vi "2.Gamepad.vi"() -> ()   [LabVIEW 2011]
doc: "This VI show how to use the basic functions in the Input Device palette. It will show information about all the joysticks, keyboards and mice attached to the system (number of axes, buttons, pov, and the name). It will also give the current information for the first joystick attached to the system (location and button pressed). The current information for the first keyboard and mouse will also be displayed."
uses:
  <vilib>/Utility/inputDevices.llb/closeJoystick.vi
  <vilib>/Utility/inputDevices.llb/joystickAcquire.vi
panel:
  out "Motor (scaled)":u64
  out "Steer (scaled)":i32
  in  "?":enum32{"Control", "Check Control"}(tab)
  in  "Steering":u8(slide)=128 scale=0.0..255.0
  in  "Motor Speed":u8(slide)=128 scale=0.0..255.0
  in  "Destination Id":u8=7
  in  "Control Mode":enum16{"Manual", "GamePad"}(ring)
  out "WriteSF Error":errorcluster
  out "OpenSF Error":errorcluster
  out "Y-axis":i32
  out "X-axis":i32
  out "Button 12":bool
  out "Button 13":bool
  out "Button 14":bool
  out "Button 15":bool
  out "X-axis":i32
  out "Y-axis":i32
  out "Value":i32
  out "Button 10":bool
  out "Button 11":bool
  out "Button 5":bool
  out "Button 6":bool
  out "POV":i32
  in  "Message":string="LabVIEW was unable\nto detect a joystick."
  in  "Button":string="Continue"
  # "Left"
  # "Right"
  # "Full Forward"
  # "Full Rverse"
  # "Left Top"
  # "Right Top"
  # "Left Buttom"
  # "Right Buttom"
  # "8-way D-pad"
  # "Left Joystick"
  # "Right Joystick"
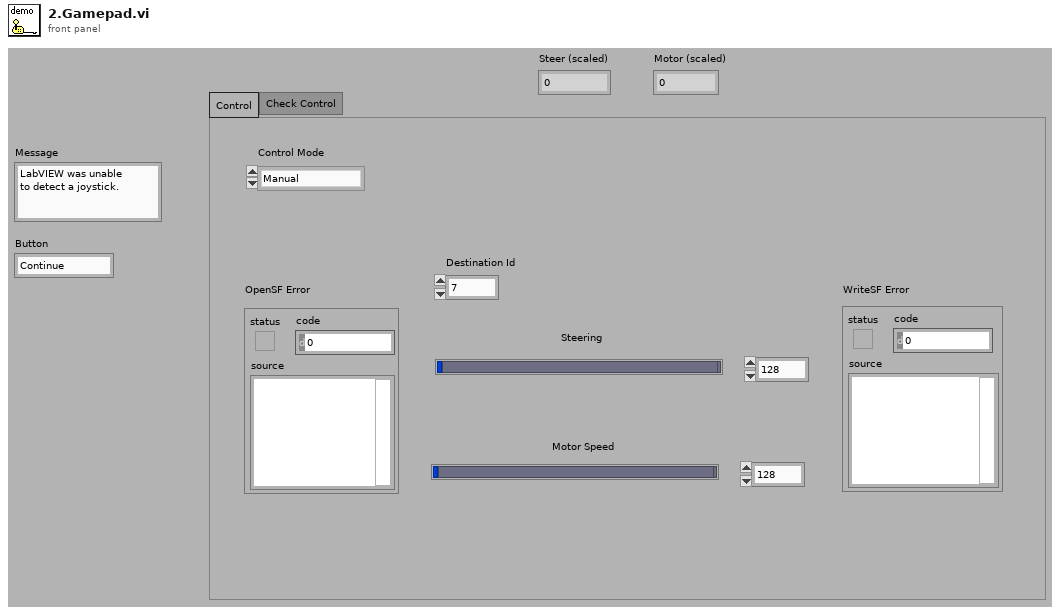
[diagram p1: front panel]
types:
  T1 = cluster{"X axis":i32, "Y axis":i32, "Z axis":i32, "X axis rotation":i32, "Y axis rotation":i32, "Z axis rotation":i32, "U axis":i32, "V axis":i32}
  T2 = cluster{"button 1":bool, "button 2":bool, "button 3":bool, "button 4":bool, "button 5":bool, "button 6":bool, "button 7":bool, "button 8":bool, "button 9":bool, "button 10":bool, "button 11":bool, "button 12":bool, "button 13":bool, "button 14":bool, "button 15":bool, "button 16":bool, "button 17":bool, "button 18":bool, "button 19":bool, "button 20":bool, "button 21":bool, "button 22":bool, "button 23":bool, "button 24":bool, "button 25":bool, "button 26":bool, "button 27":bool, "button 28":bool, "button 29":bool, "button 30":bool, "button 31":bool, "button 32":bool}
  T3 = cluster{"pov 1":i32, "pov 2":i32, "pov 3":i32, "pov 4":i32}
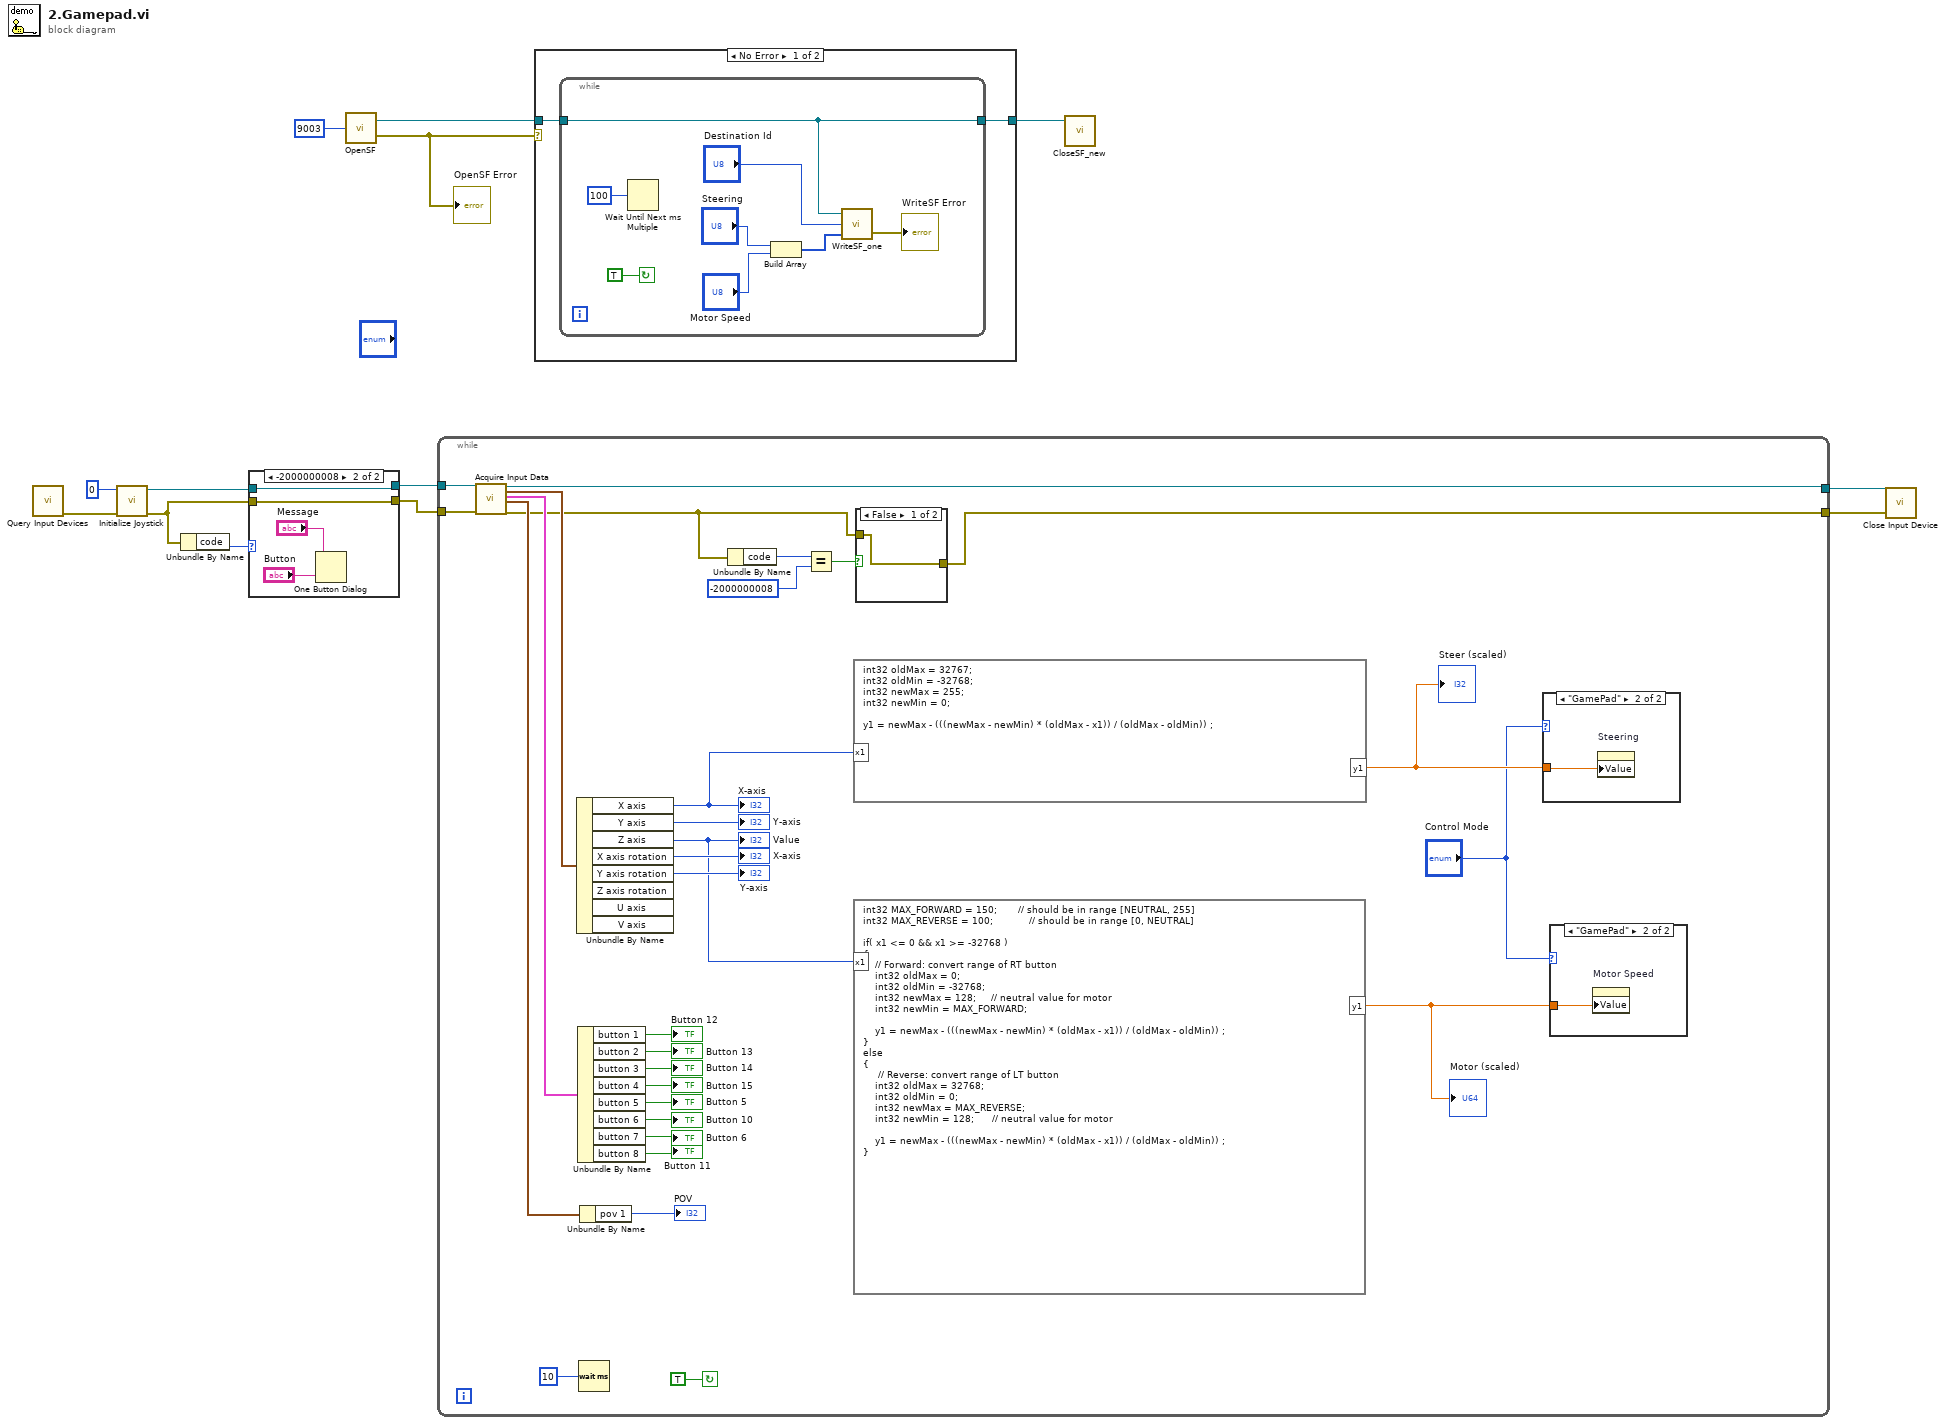
[diagram p0: block diagram]
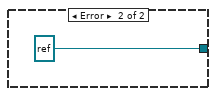
[diagram p2: hidden frame]
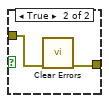
[diagram p6: hidden frame]
diagram:
  n1 = call <vilib>:"Query Input Devices.vi"() -> ("error out"=w13:errorcluster)  [unwired: 1 in, 10 out]
  n2 = call <vilib>:"Initialize Joystick.vi"("error in (no error)"=w13, "device index"=0) -> ("error out"=w7:errorcluster, "device ID"=w8:refnum<k1>)  [unwired: 8 out]
  n3 = Unbundle By Name(w7) -> ("code"=w9:i32)
  n4 = case shown="-2000000008" w9 {
    tunnel: w7 -> [w15 w17]
    tunnel: [w15 w17] -> w6
    tunnel: w8 -> [w14 w16]
    tunnel: [w14 w16] -> w5
    frame 0, Default {
    }
    frame -2000000008 {
      n5 = One Button Dialog(message="Message", button name ("OK")="Button") -> ()  [unwired: 1 out]
    }
  }
  n6 = call "OpenSF.vi"("Port number"=u16 9003 ("Port number\nactuators")) -> ("connection ID"=w2:refnum<k5>, "Error out"=w3:errorcluster)
  "OpenSF Error" <- w3
  n7 = while {
    tunnel: [w39] -> w11
    tunnel: [w43] -> w12
    tunnel: w6 -> [w37]
    tunnel: w5 -> [w36]
    stop <- TRUE continue-if-true
    n8 = call-poly <vilib>:"Acquire Input Data.vi"("device ID"=w36, "error in (no error)"=w37) -> ("device ID"=w43:refnum<k1>, "axis info"=w49:T1, "button info"=w47:T2, "direction info"=w46:T3, "error out"=w38:errorcluster)  [unwired: 13 out]
    n9 = Unbundle By Name(w49) -> ("X axis"=w26:i32, "Y axis"=→"Y-axis":i32, "Z axis"=w20:i32, "X axis rotation"=→"X-axis":i32, "Y axis rotation"=→"Y-axis":i32)  [unwired: 3 out]
    "X-axis" <- w26
    "Value" <- w20
    n10 = Unbundle By Name(w47) -> ("button 1"=→"Button 12":bool, "button 2"=→"Button 13":bool, "button 3"=→"Button 14":bool, "button 4"=→"Button 15":bool, "button 5"=→"Button 5":bool, "button 6"=→"Button 10":bool, "button 7"=→"Button 6":bool, "button 8"=→"Button 11":bool)
    n11 = Wait (ms)(milliseconds to wait=u32 10) -> ()  [unwired: 1 out]
    n12 = Unbundle By Name(w46) -> ("pov 1"=→"POV":i32)
    n13 = Unbundle By Name(w38) -> ("code"=w42:i32)
    n14 = Equal?(x=w42, y=-2000000008) -> (x = y?=w40:bool)
    n15 = formula code="int32 oldMax = 32767;\nint32 oldMin = -32768;\nint32 newMax = 255; \nint32 newMin = 0;  \n\ny1 = newMax - (((newMax - newMin) * (oldMax - x1)) / (oldMax - oldMin)) ;"("x1"=w26) -> ("y1"=w25:dbl)
    "Steer (scaled)" <- w25
    n16 = formula code="int32 MAX_FORWARD = 150;       // should be in range [NEUTRAL, 255]\nint32 MAX_REVERSE = 100;            // should be in range [0, NEUTRAL]\n\nif( x1 <= 0 && x1 >= -32768 )\n{\n    // Forward: convert range of RT button\n    int32 oldMax = 0;\n    int32 oldMin = -32768;\n    int32 newMax = 128;     // neutral value for motor\n    int32 newMin = MAX_FORWARD;    \n\n    y1 = newMax - (((newMax - newMin) * (oldMax - x1)) / (oldMax - oldMin)) ;\n}\nelse\n{\n     // Reverse: convert range of LT button\n    int32 oldMax = 32768;\n    int32 oldMin = 0;\n    int32 newMax = MAX_REVERSE;  \n    int32 newMin = 128;      // neutral value for motor\n\n    y1 = newMax - (((newMax - newMin) * (oldMax - x1)) / (oldMax - oldMin)) ;\n}"("x1"=w20) -> ("y1"=w22:dbl)
    "Motor (scaled)" <- w22
    n17 = case shown="False" w40 {
      tunnel: w38 -> [w52 w54]
      tunnel: [w52 w53] -> w39
      frame False {
      }
      frame True {
        n18 = call <vilib>:"Clear Errors.vi"("error in (no error)"=w54) -> ("error out"=w53:errorcluster)  [unwired: 6 out]
      }
    }
    n19 = case shown="\"GamePad\"" "Control Mode" {
      tunnel: w25 -> [_ w51]
      frame "Manual", Default {
      }
      frame "GamePad" {
        n20 = property on="Steering" class="Slide (strict)"("Value"=w51) -> ()  [unwired: 2 in, 2 out]
      }
    }
    n21 = case shown="\"GamePad\"" "Control Mode" {
      tunnel: w22 -> [_ w50]
      frame "Manual", Default {
      }
      frame "GamePad" {
        n22 = property on="Motor Speed" class="Slide (strict)"("Value"=w50) -> ()  [unwired: 2 in, 2 out]
      }
    }
  }
  n23 = case shown="No Error" w3 {
    tunnel: w2 -> [w56 _]
    tunnel: [w55 refnum<k5> refnum ("connection ID")] -> w1
    frame No Error {
      n24 = while {
        tunnel: w56 -> [w60]
        tunnel: [w60] -> w55
        stop <- TRUE continue-if-true
        n25 = Wait Until Next ms Multiple(millisecond multiple=u32 100) -> ()  [unwired: 1 out]
        n26 = Build Array("Steering", "Motor Speed") -> (w58:u8[])
        n27 = call "WriteSF_one.vi"("payload"=w58, "destination ID"="Destination Id", "connection ID in"=w60) -> ("error out"=→"WriteSF Error":errorcluster)  [unwired: 1 out]
      }
    }
    frame Error {
    }
  }
  n28 = call "CloseSF_new.vi"("connection ID"=w1) -> ()  [unwired: 2 in]
  n29 = call-poly <vilib>:"Close Input Device.vi"("error in (no error)"=w11, "device ID"=w12) -> ()  [unwired: 9 out]
